vi "Day 1 task 1.vi"() -> ()   [LabVIEW 2022 SP3]
panel:
  out "max value":i32
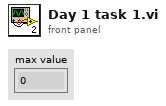
[diagram p1: front panel]
diagram:
  (unwired) "1000\n2000\n3000\n\n4000\n\n5000\n6000\n\n7000\n8000\n9000\n\n10000"
  n1 = Spreadsheet String To Array(delimiter (Tab)="\n\n", format string="%s", spreadsheet string="8462\n6981\n3714\n4409\n8186\n3614\n2218\n7558\n6702\n\n2947\n4727\n6396\n5718\n2361\n1970\n1583\n2816\n2995\n6914\n4313\n1401\n\n1643\n7815\n2162\n8841\n7671\n\n5740\n5471\n4838\n2281\n2784\n4587\n1497\n2074\n1161\n4388\n2233\n4795\n2011\n5438\n\n14064\n9646\n2537\n\n2064\n2833\n1164\n14379\n\n6008\n4327\n4709\n5412\n2745\n5680\n5322\n4375\n4064\n4822\n6523\n6824\n6822\n\n12100\n24791\n18239\n\n9704\n8218\n9949\n3078\n9407\n3732\n4281\n6727\n\n9833\n2549\n5042\n7053\n6116\n9624\n5393\n8359\n\n4195\n7869\n15434\n6997\n5776\n\n2487\n7843\n2739\n5227\n4088\n6281\n7078\n4291\n5461\n4838\n7936\n\n5449\n5754\n4685\n7642\n7244\n4912\n\n4020\n18761\n17710\n8736\n\n6204\n1295\n3812\n5078\n4627\n3818\n4351\n5202\n2542\n2728\n303...", array type (2D Dbl)=string[] []) -> (array=w6:string[])
  n2 = for {
    tunnel: w6 -> [w11] mode=indexing
    tunnel: [w8] -> w4 mode=indexing
    n3 = Spreadsheet String To Array(delimiter (Tab)="\n", format string="%d", spreadsheet string=w11, array type (2D Dbl)=i32[] []) -> (array=w9:i32[])
    n4 = Add Array Elements(numeric array=w9) -> (sum=w8:i32)
  }
  n5 = Array Max & Min(array=w4) -> (max value=→"max value":i32)  [unwired: 3 out]
